vi "bronkhorst_reg.vi"(0 "SP":dbl caption="setpoint" step=0.01 format="%.2f", 1 "PV":dbl step=0.01 format="%.2f", 2 "PV_State":T1, 3 "Y":dbl step=0.01 format="%.2f", 4 "Y_State":T1, 6 "Y_Set":T3={"Y_HSw"=1, "Y_HSetState"=enum."auto", "Y_ASetState"=enum."auto", "Y_DSetState"=enum."auto"} {"Y_HSw" max=2 step=1}, 7 "controls Y":cluster{"Y_H":dbl, "Y_A":dbl, "Y_D":dbl} {"Y_H" format="%.2f"; "Y_D" format="%#_13g"; "Y_A" format="%#_13g"}, 8 "Z":T4, 9 "control param":T7={"proportional gain (Kc)"=1.0, "integral time (Ti, s)"=10.0, "derivative time (Td, s)"=1.0, "output high"=100.0, "output high start"=40.0, "output high stop"=40.0, "alr value"=0.0, "output low"=0.0, "output rate (EGU/s)"=5.0, "setpoint max"=100.0, "setpoint rate (EGU/min)"=10.0, "stop rate (EGU/min)"=5.0} {"setpoint max" format="%.2f"; "stop rate (EGU/min)" min=0.001 format="%.2f"; "setpoint rate (EGU/min)" min=0.001 format="%.2f"; "output high stop" format="%.2f"; "output high start" format="%.2f"; "output rate (EGU/s)" min=0.001 format="%.2f"; "output low" format="%.2f"; "alr value" format="%.2f"; "output high" format="%.2f"; "derivative time (Td, s)" format="%.3f"; "integral time (Ti, s)" format="%.3f"; "proportional gain (Kc)" format="%.3f"}, 10 "XB24 (F)":bool) -> (13 "YB":bool, 14 "Y_State":T5={"Y_Source"=enum."local disabled", "Y_SetState"=enum."auto", "SP_Set"=0.0, "SP"=0.0, "PV"=0.0, "PV_State"={"code"=0, "visible"=FALSE, "color"=0}, "Y_preSet"=0.0, "Y_Set"=0.0, "Y"=0.0, "Y_State"={"code"=0, "visible"=FALSE, "color"=0}, "YB"=FALSE} {"Y" format="%.2f"; "Y_preSet" format="%.2f"; "SP" step=0.01 format="%.2f"; "Y_Set" format="%.2f"; "PV" step=0.01 format="%.2f"; "SP_Set" step=0.01 format="%.2f"}, 15 "Y":dbl format="%.2f", 17 "T":u32, 18 "End":bool)   [LabVIEW 2019, in "control.lvlib"]
uses:
  control.lvlib
  ctl/control param.ctl
  ctl/Y.ctl
  ctl/Y_source.ctl
  ctl/Y_state.ctl
  Inputs/Ctl/Parameter State short.ctl
  ctl/Z_State.ctl
  ctl/SpLim_State.ctl
  PID Output Rate Limiter.vi
  PID Output Rate Limiter Ext.vi
  PID Timing Estimation Ext.vi
  PID Timing Estimation.vi
  Userlib.lvlib
  Inputs/Inputs.lvlib
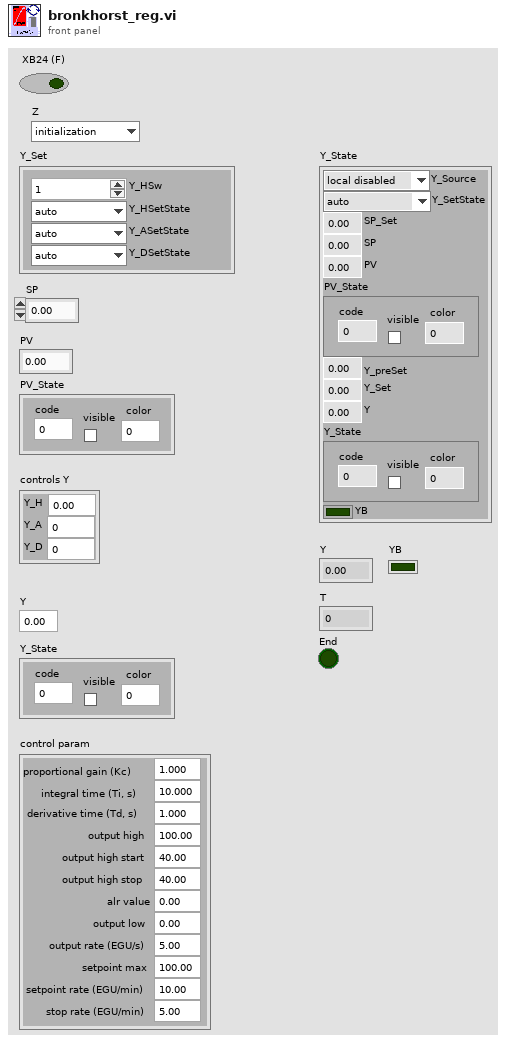
[diagram p1: front panel]
types:
  T1 = typedef "Inputs.lvlib/Parameter State short.ctl" = cluster{"code":i32, "visible":bool, "color":u32}
  T2 = typedef "control.lvlib/Y_state.ctl" = enum8{"initialize", "alarm", "min", "stop", "hand", "auto", "max"}
  T3 = cluster{"Y_HSw":u32, "Y_HSetState":T2, "Y_ASetState":T2, "Y_DSetState":T2}
  T4 = typedef "control.lvlib/Z_State.ctl" = enum8{"initialization", "alarm", "disabled", "not ready", "stop ready", "reserv", "switched off", "reserv2", "switched on", "check", "on min", "decrease out", "on", "increase out", "on max"}
  T5 = typedef "control.lvlib/Y.ctl" = cluster{"Y_Source":T6, "Y_SetState":T2, "SP_Set":dbl, "SP":dbl, "PV":dbl, "PV_State":T1, "Y_preSet":dbl, "Y_Set":dbl, "Y":dbl, "Y_State":T1, "YB":bool}
  T6 = typedef "control.lvlib/Y_source.ctl" = enum8{"initialize", "local disabled", "local hand", "hand", "auto", "dist"}
  T7 = typedef "control.lvlib/control param.ctl" = cluster{"proportional gain (Kc)":dbl, "integral time (Ti, s)":dbl, "derivative time (Td, s)":dbl, "output high":dbl, "output high start":dbl, "output high stop":dbl, "alr value":dbl, "output low":dbl, "output rate (EGU/s)":dbl, "setpoint max":dbl, "setpoint rate (EGU/min)":dbl, "stop rate (EGU/min)":dbl}
  T8 = typedef "control.lvlib/SpLim_State.ctl" = enum8{"initialization", "stop", "decrease", "increase"}
  T9 = typedef "control.lvlib/PID param.ctl" = cluster{"proportional gain (Kc)":dbl, "integral time (Ti, s)":dbl, "derivative time (Td, s)":dbl, "output high":dbl, "alr value":dbl, "output low":dbl, "output rate (EGU/s)":dbl, "dt (s)":dbl}
  T10 = enum8{"alarm", "min", "stop", "hand", "auto", "max"}
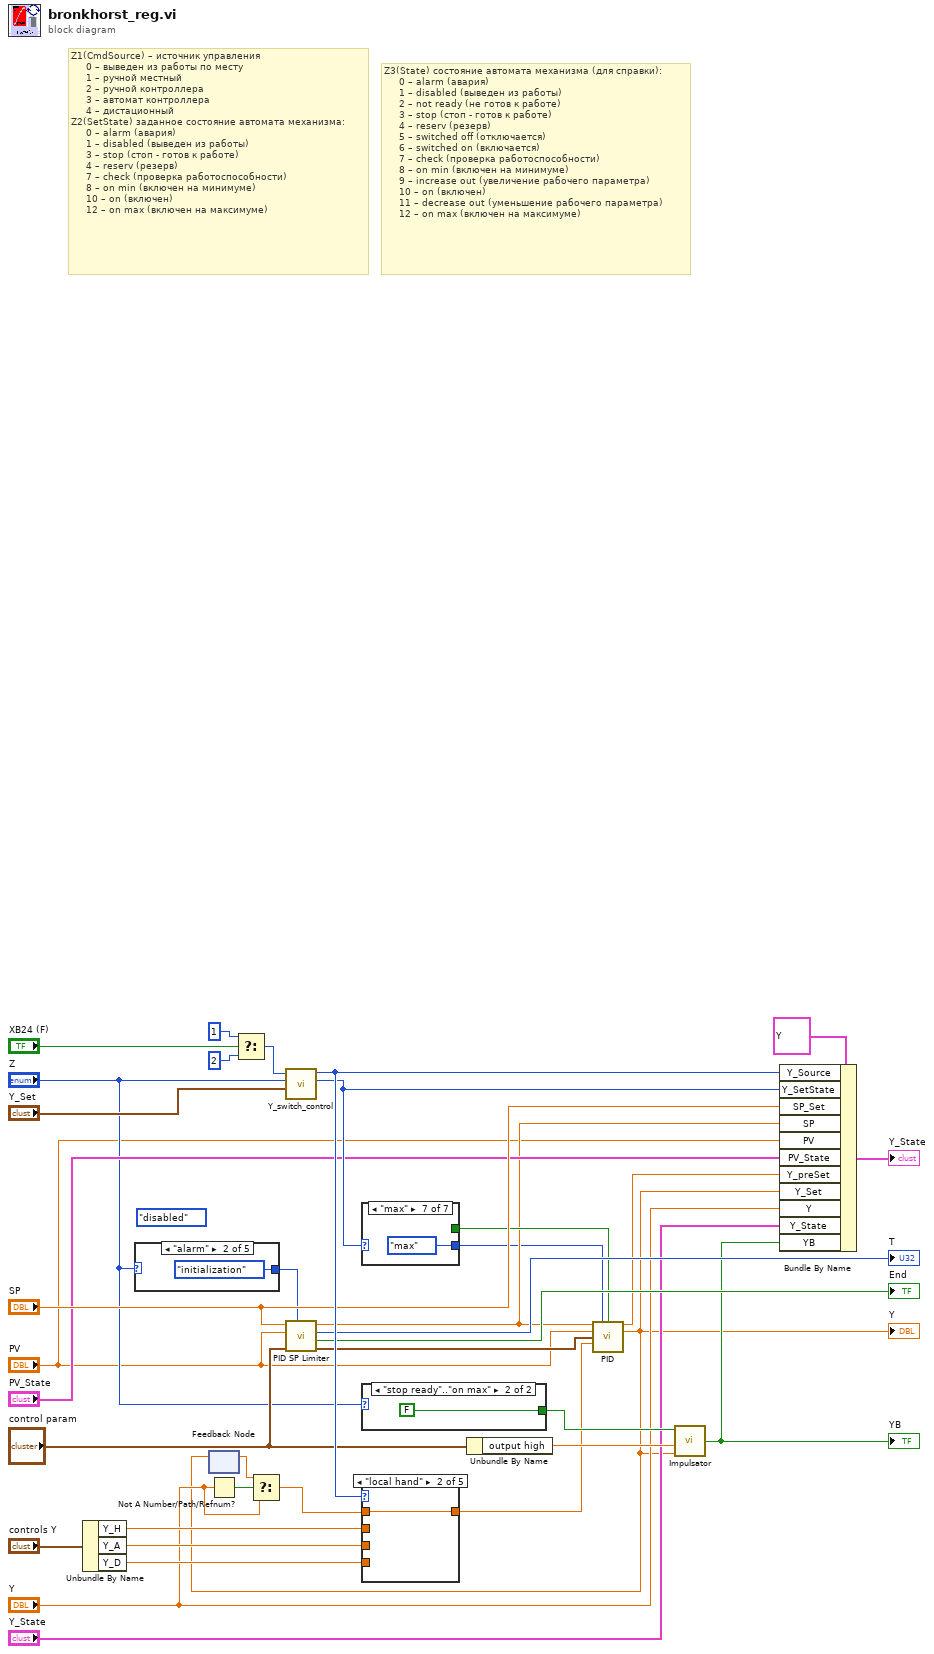
[diagram p0: block diagram]
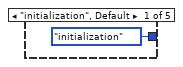
[diagram p2: hidden frame]
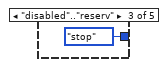
[diagram p3: hidden frame]
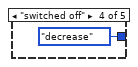
[diagram p4: hidden frame]
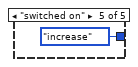
[diagram p5: hidden frame]
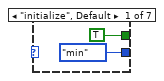
[diagram p6: hidden frame]
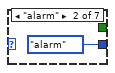
[diagram p7: hidden frame]
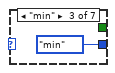
[diagram p8: hidden frame]
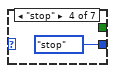
[diagram p9: hidden frame]
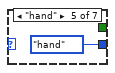
[diagram p10: hidden frame]
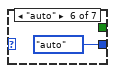
[diagram p11: hidden frame]
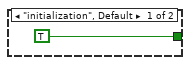
[diagram p12: hidden frame]
diagram:
  (unwired) Z_State."disabled" ("Z")
  # "Z1(CmdSource) – источник управления\n     0 – выведен из работы по месту\n     1 – ручной местный\n     2 – ручной контроллера\n     3 – автомат контроллера\n     4 – дистационный\nZ2(SetState) заданное состояние автомата механизма:\n     0 – alarm (авария)\n     1 – disabled (выведен из работы)\n     3 – stop (стоп - готов к работе)\n     4 – reserv (резерв)\n     7 – check (проверка работоспособности)\n     8 – on min (включен на минимуме)\n     10 – on (включен)\n     12 – on max (включен на максимуме)"
  # "Z3(State) состояние автомата механизма (для справки):\n     0 – alarm (авария)\n     1 – disabled (выведен из работы)\n     2 – not ready (не готов к работе)\n     3 – stop (стоп - готов к работе)\n     4 – reserv (резерв)\n     5 – switched off (отключается)\n     6 – switched on (включается)\n     7 – check (проверка работоспособности)\n     8 – on min (включен на минимуме)\n     9 – increase out (увеличение рабочего параметра)\n     10 – on (включен)\n     11 – decrease out (уменьшение рабочего параметра)\n     12 – on max (включен на максимуме)"
  n1 = Unbundle By Name("controls Y") -> ("Y_H"=w13:dbl, "Y_A"=w35:dbl, "Y_D"=w34:dbl)
  n2 = case shown="\"alarm\"" "Z" {
    tunnel: [SpLim_State."initialization" ("SpLim_State") SpLim_State."initialization" ("SpLim_State") SpLim_State."stop" ("SpLim_State") SpLim_State."decrease" ("SpLim_State") SpLim_State."increase" ("SpLim_State")] -> w20
    frame "initialization", Default {
    }
    frame "alarm" {
    }
    frame "disabled".."reserv" {
    }
    frame "switched off" {
    }
    frame "switched on" {
    }
  }
  n3 = feedback #1() -> (w9:dbl)  [unwired: 1 in]
  n4 = Not A Number/Path/Refnum?(number/path/refnum="Y") -> (NaN/Path/Refnum?=w12:bool)
  n5 = Select(t=u32 1, s="XB24 (F)", f=u32 2 ("Y_HSw")) -> (s? t:f=w31:u32)
  n6 = Select(t=w9, s=w12, f="Y") -> (s? t:f=w10:dbl)
  n7 = call "Y_switch_control.vi"("Y"="Y_Set", "Z_State"="Z", "Y_LSw (2-auto)"=w31) -> ("Y_SetState"=w28:T2, "Y_Source"=w29:T6)  [unwired: 7 in]
  n8 = call "PID SP Limiter.vi"("SpLim_State"=w20, "REG param"="control param", "PV"="PV", "SP"="SP") -> ("PID param"=w4:T9, "End"=→"End":bool, "T"=→"T":u32, "output"=w6:dbl)  [unwired: 4 in]
  n9 = case shown="\"max\"" w28 {
    tunnel: [T10."min" ("X1(SetState)") T10."alarm" ("X1(SetState)") T10."min" ("X1(SetState)") T10."stop" ("X1(SetState)") T10."hand" ("X1(SetState)") T10."auto" ("X1(SetState)") T10."max" ("X1(SetState)")] -> w5
    tunnel: [TRUE _ _ _ _ _ _] -> w8
    frame "initialize", Default {
    }
    frame "alarm" {
    }
    frame "min" {
    }
    frame "stop" {
    }
    frame "hand" {
    }
    frame "auto" {
    }
    frame "max" {
    }
  }
  n10 = case shown="\"stop ready\"..\"on max\"" "Z" {
    tunnel: [TRUE FALSE] -> w23
    frame "initialization", Default {
    }
    frame "stop ready".."on max" {
    }
  }
  n11 = case shown="\"local hand\"" w29 {
    tunnel: w13 -> [_ _ w54 _ _]
    tunnel: w10 -> [w52 w53 _ _ _]
    tunnel: w34 -> [_ _ _ _ w56]
    tunnel: [w52 w53 w54 w55 w56] -> w2
    tunnel: w35 -> [_ _ _ w55 _]
    frame "local disabled", Default {
    }
    frame "local hand" {
    }
    frame "hand" {
    }
    frame "auto" {
    }
    frame "dist" {
    }
  }
  n12 = Unbundle By Name("control param") -> ("output high"=w25:dbl)
  n13 = call "PID.vi"("setpoint"=w6, "X1(SetState)"=w5, "reinitialize? (F)"=w8, "process variable"="PV", "PID param"=w4, "manual control"=w2) -> ("set output"=w7:dbl, "output"=w1:dbl)  [unwired: 7 in, 1 out]
  "Y" <- w1
  n14 = feedback-in #1(w1) -> ()
  n15 = call "Impulsator.vi"("PV"=w1, "upper limit"=w25, "Initialise"=w23) -> ("Y"=w16:bool)  [unwired: 1 in]
  "YB" <- w16
  n16 = Bundle By Name(cluster=T5 {"Y_Source"=enum."local disabled", "Y_SetState"=enum."auto", "SP_Set"=0.0, "SP"=0.0, "PV"=0.0, "PV_State"={"code"=0, "visible"=FALSE, "color"=0}, "Y_preSet"=0.0, "Y_Set"=0.0, "Y"=0.0, "Y_State"={"code"=0, "visible"=FALSE, "color"=0}, "YB"=FALSE} ("Y_State"), "Y_Source"=w29, "Y_SetState"=w28, "SP_Set"="SP", "SP"=w6, "PV"="PV", "PV_State"="PV_State", "Y_preSet"=w7, "Y_Set"=w1, "Y"="Y", "Y_State"="Y_State", "YB"=w16) -> (→"Y_State":T5)
